vi "DeleteContact.vi"(7 "LabVIEW Web Service Request":refnum<class "Web Request.lvclass">, 11 "ID":u32) -> ()   [LabVIEW 2014]
doc: "This HTTP Method VI deletes a contact from the address book data store using the ID input. It then redirects back to the contacts list."
uses:
  <vilib>/wsapi/Web Request.lvclass
  Libraries/Contact Data/Contact Data.lvlib
panel:
  # "Because this is an HTTP Method VI, LabVIEW Web Service Request is populated automatically."
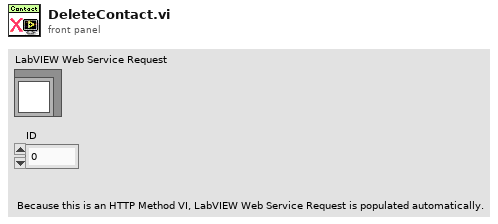
[diagram p1: front panel]
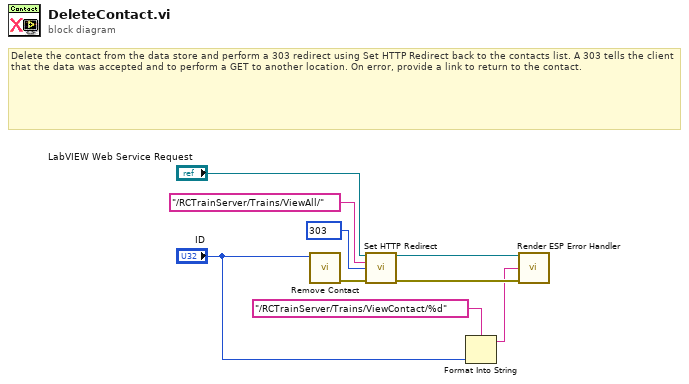
[diagram p0: block diagram]
diagram:
  w9 = 303 items=["100"=100, "101"=101, "200"=200, "201"=201, "202"=202, "203"=203, "204"=204, "205"=205, "206"=206, "300"=300, "301"=301, "302"=302, "303"=303, "304"=304, "305"=305, "306"=306, "307"=307, "400"=400, "401"=401, "402"=402, "403"=403, "404"=404, "405"=405, "406"=406, "407"=407, "408"=408, "409"=409, "410"=410, "411"=411, "412"=412, "413"=413, "414"=414, "415"=415, "416"=416, "417"=417, "500"=500, "501"=501, "502"=502, "503"=503, "504"=504, "505"=505] ("response code (307)")
  # "Delete the contact from the data store and perform a 303 redirect using Set HTTP Redirect back to the contacts list. A 303 tells the client that the data was accepted and to perform a GET to another location. On error, provide a link to return to the contact."
  n1 = call "Remove Contact.vi"("ID"="ID") -> ("error out"=w1:errorcluster)  [unwired: 10 in]
  n2 = call <vilib>:"Set HTTP Redirect.vi"("LabVIEW Web Service Request"="LabVIEW Web Service Request", "redirect URL"="/RCTrainServer/Trains/ViewAll/", "response code (307)"=w9, "error in (no error)"=w1) -> ("LabVIEW Web Service Request out"=w4:refnum<class "Web Request.lvclass">, "error out"=w5:errorcluster)  [unwired: 10 in]
  n3 = Format Into String(format string="/RCTrainServer/Trains/ViewContact/%d" ("Link"), "ID") -> (resulting string=w3:string)  [unwired: 2 in, 1 out]
  n4 = call "Render ESP Error Handler.vi"("LabVIEW Web Service Request"=w4, "Link"=w3, "error in (no error)"=w5) -> ()  [unwired: 11 in, 2 out]
